vi "Parse Response String.vi"(8 "error in (no error)":errorcluster, 10 "Response String in":string, 11 "Return Request in":T1) -> (0 "error out":errorcluster, 2 "Response String out":string, 3 "Return Request out":T1)   [LabVIEW 2017, in "SSH.lvlib"]
doc: "Parses a response string to determine if a trigger condition has occurred, and if so send out the response"
uses:
  SSH.lvlib
  Return Request Configuration.ctl
  Response Configuration.ctl
  5822de49-7e8d-462b-959c-6f44863453a5.vi
  23640ccb-d23e-4a0f-bc9c-305a9d7cbcf0.vi
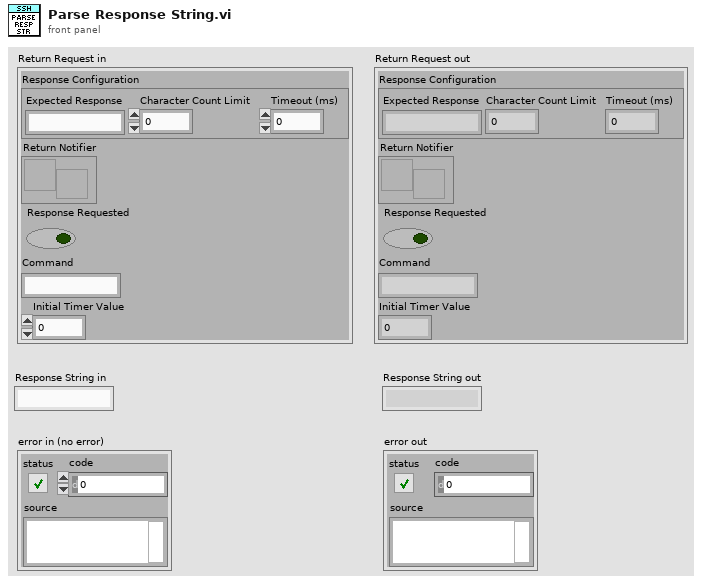
[diagram p1: front panel]
types:
  T1 = typedef "SSH.lvlib/Return Request Configuration.ctl" = cluster{"Response Configuration":T2, "Return Notifier":refnum<notifier>, "Response Requested":bool, "Command":string, "Initial Timer Value":u32}
  T2 = typedef "SSH.lvlib/Response Configuration.ctl" = cluster{"Expected Response":string, "Character Count Limit":i32, "Timeout (ms)":u32}
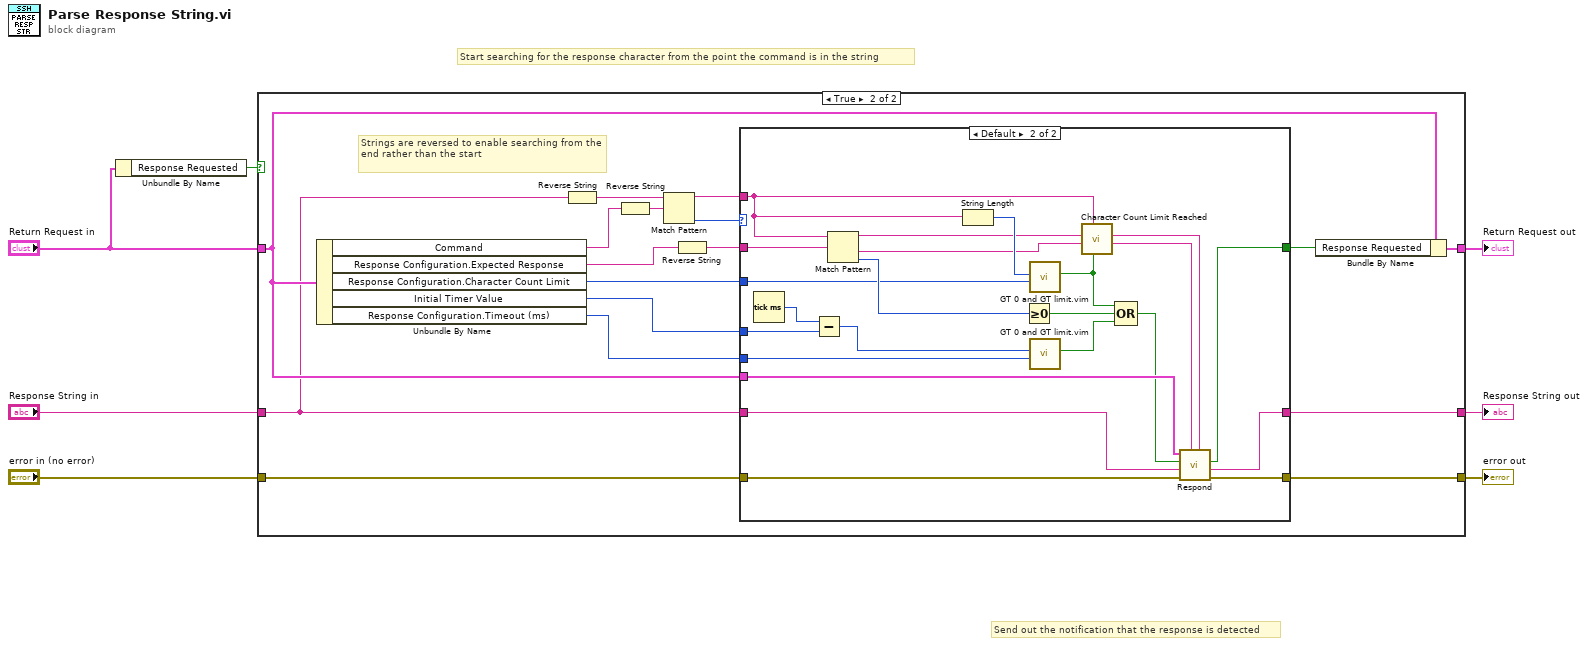
[diagram p0: block diagram]
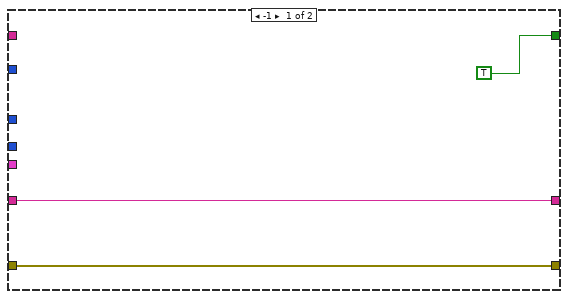
[diagram p3: hidden frame]
diagram:
  # "Send out the notification that the response is detected"
  # "Start searching for the response character from the point the command is in the string"
  n1 = Unbundle By Name("Return Request in") -> ("Response Requested"=w7:bool)
  n2 = case shown="True" w7 {
    tunnel: "Response String in" -> [w9 w20]
    tunnel: [w9 w27] -> w5
    tunnel: "error in (no error)" -> [w8 w26]
    tunnel: [w8 w25] -> w3
    tunnel: "Return Request in" -> [w10 w23]
    tunnel: [w10 w21] -> w1
    frame False {
    }
    frame True {
      # "Strings are reversed to enable searching from the end rather than the start"
      n3 = Unbundle By Name(w23) -> ("Command"=w12:string, "Response Configuration.Expected Response"=w24:string, "Response Configuration.Character Count Limit"=w13:i32, "Initial Timer Value"=w14:u32, "Response Configuration.Timeout (ms)"=w11:u32)
      n4 = Reverse String(1:w20) -> (0:w19:string)
      n5 = Reverse String(1:w12) -> (0:w18:string)
      n6 = Match Pattern(string=w19, regular expression=w18) -> (before substring=w17:string, offset past match=w15:i32)  [unwired: 1 in, 2 out]
      n7 = Reverse String(1:w24) -> (0:w16:string)
      n8 = case shown="Default" w15 {
        tunnel: [w29 w42] -> w27
        tunnel: w26 -> [w28 w52]
        tunnel: [w28 w51] -> w25
        tunnel: w23 -> [_ w50]
        tunnel: [TRUE w49] -> w22
        tunnel: w20 -> [w29 w48]
        tunnel: w17 -> [_ w31]
        tunnel: w16 -> [_ w47]
        tunnel: w14 -> [_ w45]
        tunnel: w11 -> [_ w39]
        tunnel: w13 -> [_ w40]
        frame -1 {
        }
        frame Default {
          n9 = Tick Count (ms)() -> (millisecond timer value=w46:u32)
          n10 = Subtract(x=w46, y=w45) -> (x-y=w38:u32)
          n11 = Match Pattern(string=w31, regular expression=w47) -> (before substring=w35:string, after substring=w34:string, offset past match=w53:i32)  [unwired: 1 in, 1 out]
          n12 = String Length(string=w31) -> (length=w41:i32)
          n13 = Greater Or Equal To 0?(x=w53) -> (x >= 0?=w44:bool)
          n14 = call "GT 0 and GT limit.vim"("Limit"=w40, "Count"=w41) -> ("Boolean"=w36:bool)  [unwired: 9 in]
          n15 = call "GT 0 and GT limit.vim"("Limit"=w39, "Count"=w38) -> ("Boolean"=w37:bool)  [unwired: 9 in]
          n16 = call "Character Count Limit Reached.vi"("Character Count Limit Reached"=w36, "Full String"=w31, "Response In"=w34, "Remaining string in"=w35) -> ("Response out"=w33:string, "Remaining string out"=w32:string)  [unwired: 6 in]
          n17 = Compound Arithmetic op=OR(w36, w44, w37) -> (w43:bool)
          n18 = call "Respond.vi"("Remaining String (Reversed)"=w32, "Response (Reversed)"=w33, "error in (no error)"=w52, "String buffer in"=w48, "Response triggered"=w43, "Return Request in"=w50) -> ("error out"=w51:errorcluster, "String buffer out"=w42:string, "Response Flag"=w49:bool)  [unwired: 3 in]
        }
      }
      n19 = Bundle By Name(cluster=w23, "Response Requested"=w22) -> (w21:T1)
    }
  }
  "error out" <- w3
  "Return Request out" <- w1
  "Response String out" <- w5
